vi "Check moving.vi"(8 "error in (no error)":errorcluster, 10 "tracking code":string, 11 "Motor in":refnum<class "Motor.lvclass">) -> (0 "error out":errorcluster, 2 "moving":bool, 3 "Motor out":refnum<class "Motor.lvclass">)   [LabVIEW 2018, in "Motor.lvclass"]
uses:
  Motor.lvclass
  Motor.lvclass/Motor.ctl
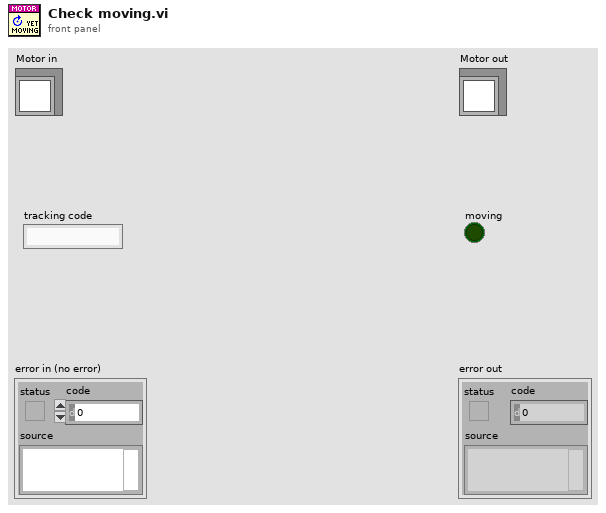
[diagram p1: front panel]
types:
  T1 = cluster{"mode":string, "condition":string, "position":string, "pos_name":string, "pos_id":string}
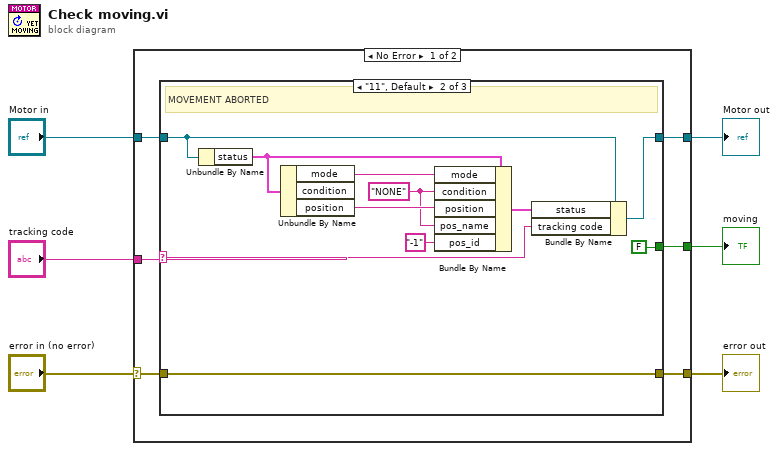
[diagram p0: block diagram]
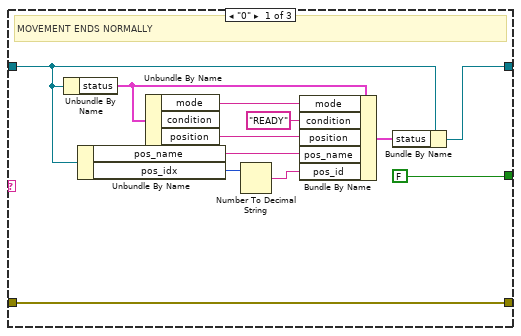
[diagram p2: hidden frame]
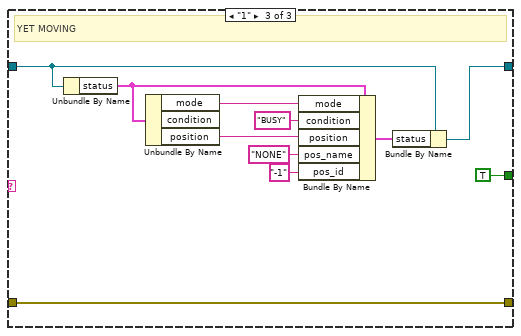
[diagram p3: hidden frame]
diagram:
  n1 = case shown="No Error" "error in (no error)" {
    selector: "error in (no error)" -> [w9 w47]
    tunnel: [w8 w47] -> w5
    tunnel: [w7 w48] -> w3
    tunnel: "Motor in" -> [w10 w48]
    tunnel: "tracking code" -> [w12 _]
    tunnel: [w11 _] -> w1
    frame No Error {
      n2 = case shown="\"11\", Default" w12 {
        selector: w12 -> [_ w25 _]
        tunnel: [FALSE FALSE TRUE] -> w11
        tunnel: w10 -> [w14 w29 w39]
        tunnel: w9 -> [w24 w35 w45]
        tunnel: [w24 w35 w45] -> w8
        tunnel: [w13 w28 w38] -> w7
        frame "0" {
          # "MOVEMENT ENDS NORMALLY"
          n3 = Unbundle By Name(w14) -> ("status"=w23:T1)
          n4 = Unbundle By Name(w14) -> ("pos_name"=w19:string, "pos_idx"=w21:i32)
          n5 = Unbundle By Name(w23) -> ("mode"=w22:string, "position"=w17:string)  [unwired: 1 out]
          n6 = Number To Decimal String(number=w21) -> (decimal integer string=w20:string)  [unwired: 1 in]
          n7 = Bundle By Name(cluster=w23, "mode"=w22, "condition"="READY", "position"=w17, "pos_name"=w19, "pos_id"=w20) -> (w15:T1)
          n8 = Bundle By Name(cluster=w14, "status"=w15) -> (w13:refnum<class "Motor.lvclass">)
        }
        frame "11", Default {
          w27 = "NONE" ("condition")
          # "MOVEMENT ABORTED"
          n9 = Unbundle By Name(w29) -> ("status"=w34:T1)
          n10 = Unbundle By Name(w34) -> ("mode"=w33:string, "position"=w32:string)  [unwired: 1 out]
          n11 = Bundle By Name(cluster=w34, "mode"=w33, "condition"=w27, "position"=w32, "pos_name"=w27, "pos_id"="-1") -> (w30:T1)
          n12 = Bundle By Name(cluster=w29, "status"=w30, "tracking code"=w25) -> (w28:refnum<class "Motor.lvclass">)
        }
        frame "1" {
          # "YET MOVING"
          n13 = Unbundle By Name(w39) -> ("status"=w44:T1)
          n14 = Unbundle By Name(w44) -> ("mode"=w43:string, "position"=w41:string)  [unwired: 1 out]
          n15 = Bundle By Name(cluster=w44, "mode"=w43, "condition"="BUSY", "position"=w41, "pos_name"="NONE" ("condition"), "pos_id"="-1" ("condition")) -> (w40:T1)
          n16 = Bundle By Name(cluster=w39, "status"=w40) -> (w38:refnum<class "Motor.lvclass">)
        }
      }
    }
    frame Error {
    }
  }
  "error out" <- w5
  "Motor out" <- w3
  "moving" <- w1
